vi "Memory.vi"(6 "Put":bool, 8 "error in (no error)":errorcluster, 11 "SECS Data Class in":refnum<class "SECS Data Class.lvclass">) -> (0 "error out":errorcluster, 3 "SECS Data Class out":refnum<class "SECS Data Class.lvclass">)   [LabVIEW 2020, in "SECS Communication.lvlib" / "SECS Data Class.lvclass"]
uses:
  SECS Data Class.lvclass
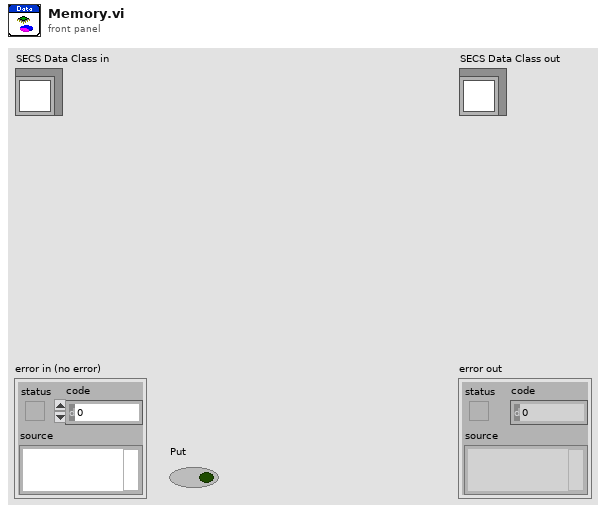
[diagram p1: front panel]
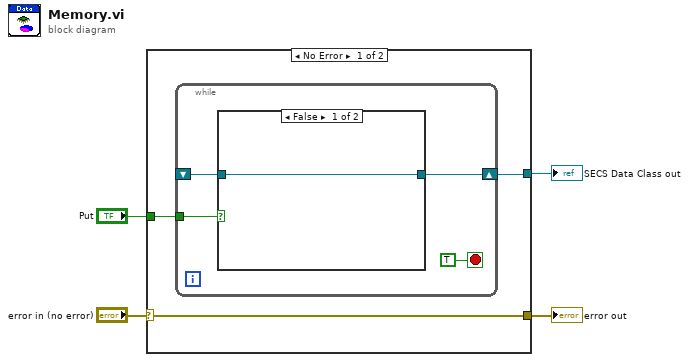
[diagram p0: block diagram]
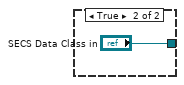
[diagram p2: hidden frame]
diagram:
  n1 = case shown="No Error" "error in (no error)" {
    selector: "error in (no error)" -> [w6 w14]
    tunnel: "Put" -> [w7 _]
    tunnel: [w6 w14] -> w1
    tunnel: [w5 _] -> w2
    frame No Error {
      n2 = while {
        shift-right: [w10] -> w5
        shift-left: _ -> [w9]
        tunnel: w7 -> [w11]
        stop <- TRUE stop-if-true
        n3 = case shown="False" w11 {
          tunnel: [w12 "SECS Data Class in"] -> w10
          tunnel: w9 -> [w12 _]
          frame False {
          }
          frame True {
          }
        }
      }
    }
    frame Error {
    }
  }
  "error out" <- w1
  "SECS Data Class out" <- w2
